vi "State Logic.vi"(0 "TLB' data in":refnum<class "Synchronize AWS S3 Content TLB`.lvclass">, 1 "process state logic enable":bool, 5 "trigger queue in":refnum<queue>, 7 "action queue in":refnum<queue>, 11 "error in":errorcluster) -> (4 "TLB' data out":refnum<class "Synchronize AWS S3 Content TLB`.lvclass">, 15 "error out":errorcluster)   [LabVIEW 2026, in "Synchronize AWS S3 Content.lvlib" / "Synchronize AWS S3 Content TLB`.lvclass"]
doc: "Control process for TLB' template.\n\n<B>Input Parameters</B>\n\n<B>TLB' data in</B> is the templates' private data.\n\n<B>process state logic enable</B> enable state logic change.\n\n<B>trigger queue in</B> is a reference to a queue. Use the Create Trigger Queue function to obtain a queue reference. \n\n<B>action queue in</B> is a reference to a queue. Use the Create Action Queue function to obtain a queue reference. \n\n<B>timeout (ms)</B> queue timeout.\n\n<B>error in</B> describes error conditions that occur before this node runs. This input provides standard error in functionality.\n\n<B>Output Parameters</B>\n\n<B>TLB' data out</B> is the templates' private data.\n\n<B>error out</B> contains error information. This output provides standard error out functionality."
uses:
  Synchronize AWS S3 Content TLB`.lvclass
  Application Components/Trigger API/System Trigger Element.ctl
  Application Components/Trigger API/System Trigger.ctl
  Core Components/Actions/System Action Element.ctl
  Synchronize AWS S3 Content TLB`.lvclass/Synchronize AWS S3 Content TLB`.ctl
  State.ctl
  Core Components/Error Handler/TLB` Error Handler.lvclass/TLB` Error Handler.ctl
  Core Components/Error Handler/accessors/Get Action Causing Error.vi
  Core Components/Error Handler/accessors/Get Originating State.vi
  Core Components/Error Handler/accessors/Get Destination State.vi
  Core Components/Error Handler/accessors/Get Executed System Actions.vi
  Core Components/Error Handler/accessors/Get Remaing System Actions.vi
  Core Components/Error Handler/Core/actions/support/Error FLUSH-LOG-DIALOG.vi
  Core Components/Error Handler/Core/actions/support/Error FLUSH-DIALOG.vi
  Application Components/Trigger API/Synchronize AWS S3 Content Trigger API.lvlib
  Core Components/Error Handler/TLB` Error Handler.lvclass
  Core Components/Actions/Actions.lvlib
  Synchronize AWS S3 Content.lvlib
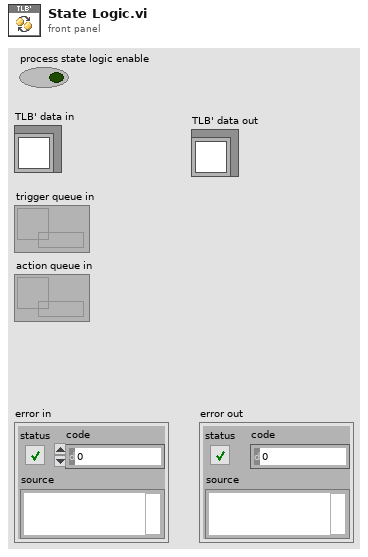
[diagram p1: front panel]
types:
  T1 = typedef "Synchronize AWS S3 Content.lvlib/Synchronize AWS S3 Content TLB`.lvclass/State.ctl" = enum16{"<Startup>", "Idle", "Initiating Configuration", "Validating Commands", "Executing Synchronization", "Validation", "<Shutdown>", "<Error>"}
  T2 = typedef "Synchronize AWS S3 Content.lvlib/Synchronize AWS S3 Content Trigger API.lvlib/System Trigger.ctl" = enum16{"<None>", "<Return to Safe State Actions>", "<Cache User Parameters>", "<Close Application>", "<Error>"}
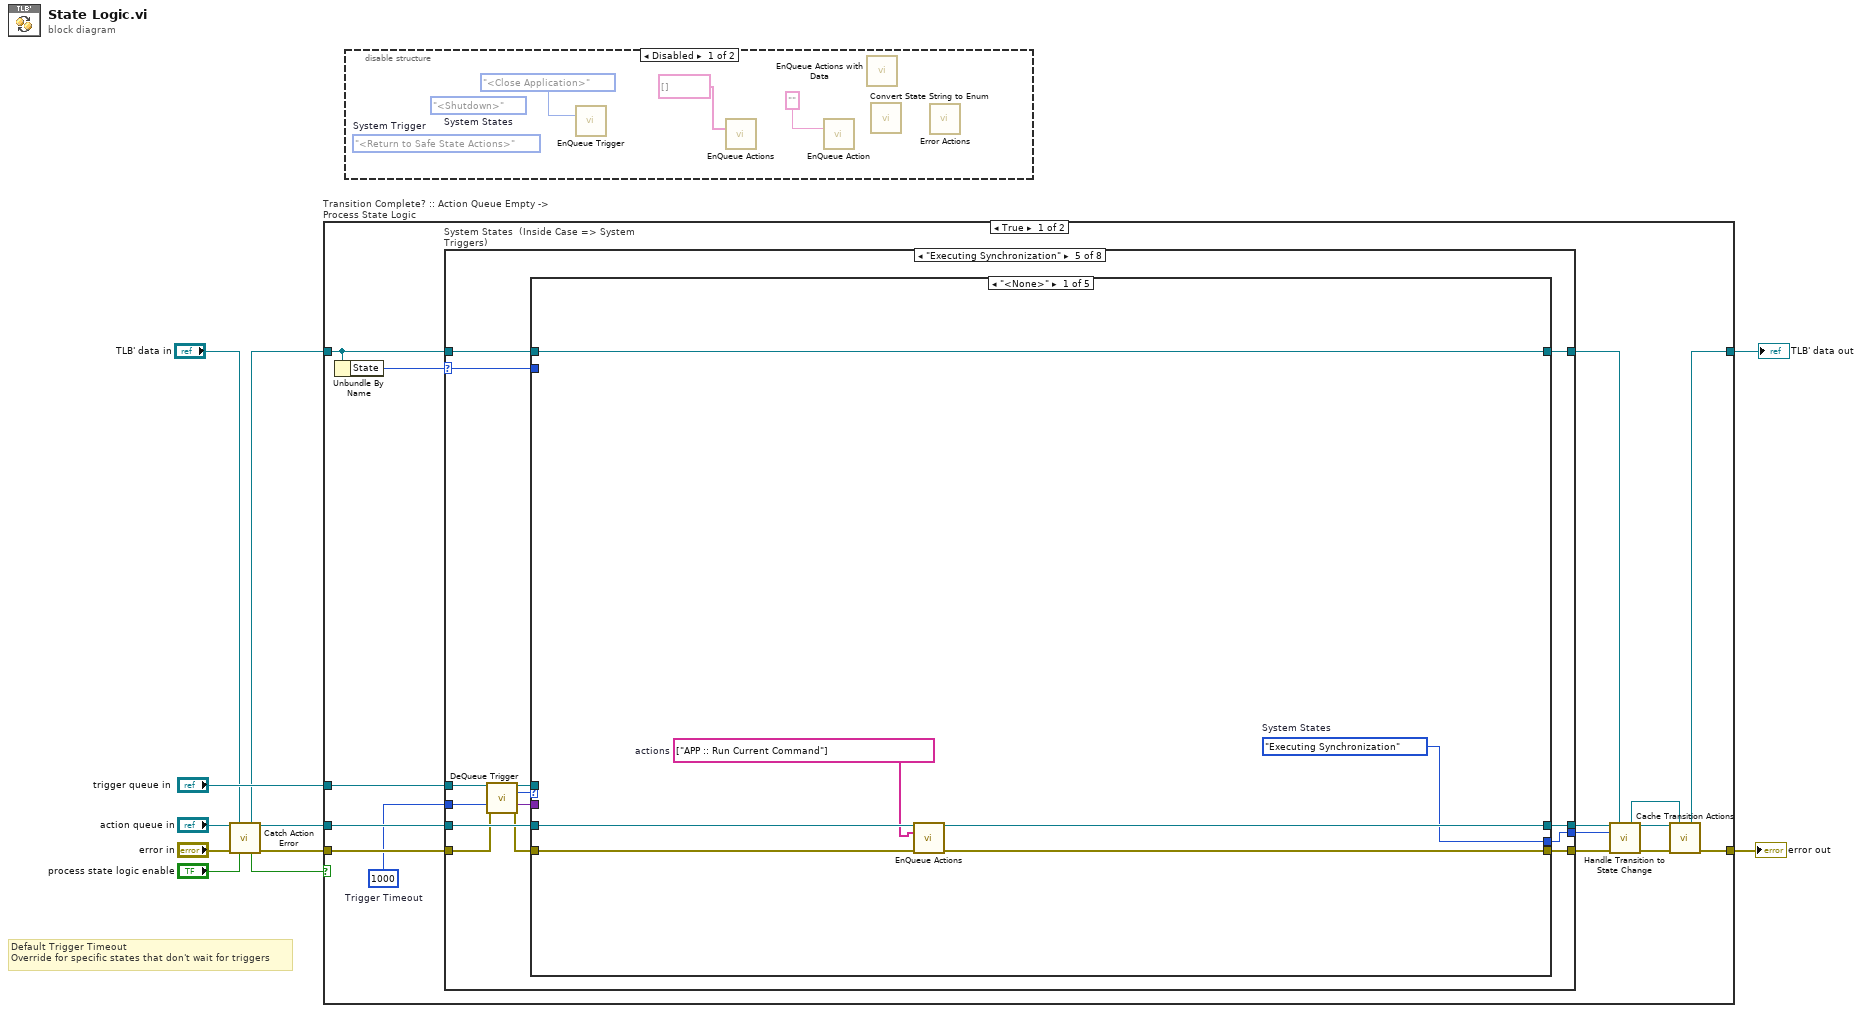
[diagram p0: block diagram]
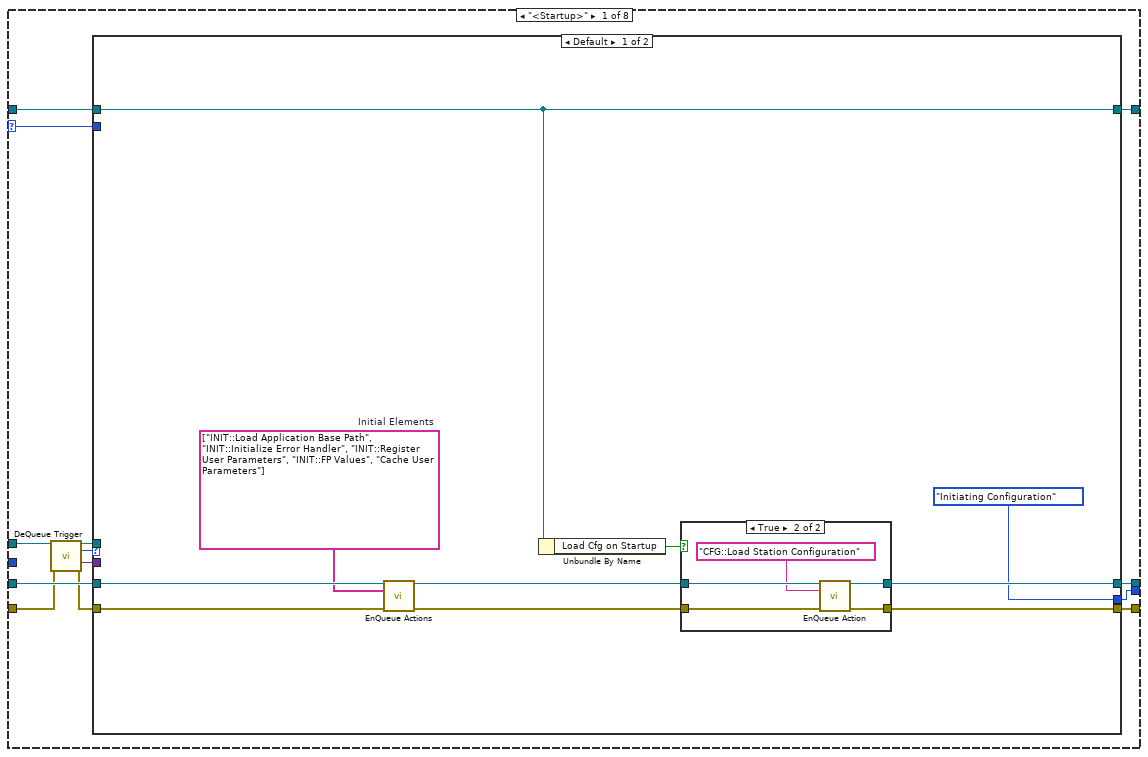
[diagram p3: hidden frame]
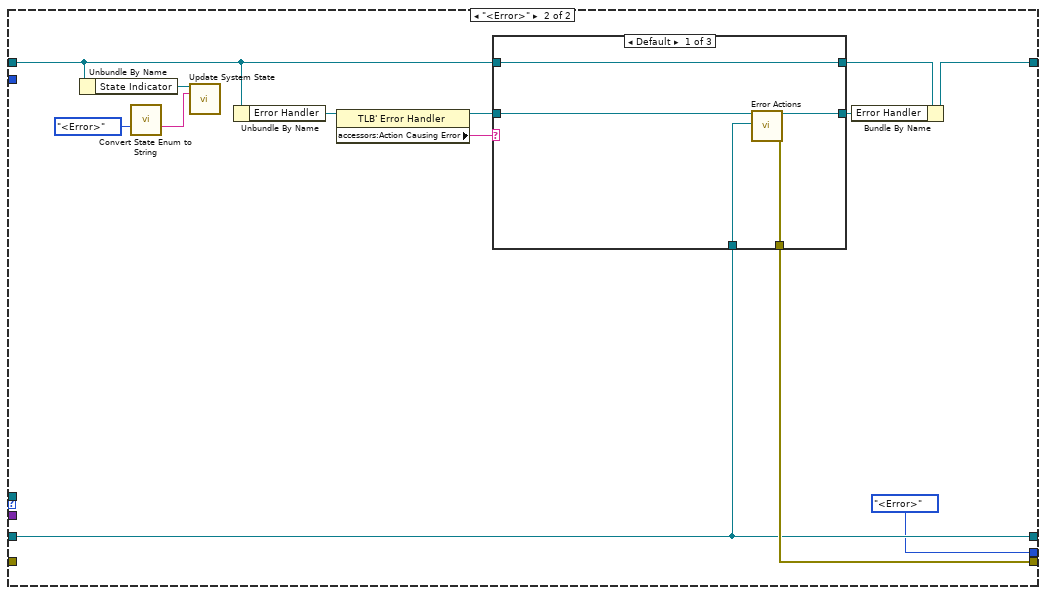
[diagram p5: hidden frame]
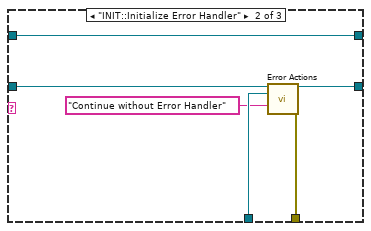
[diagram p6: hidden frame]
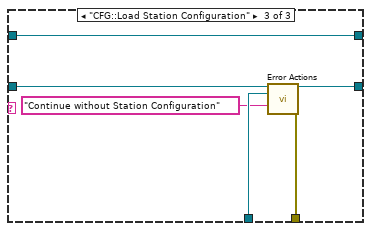
[diagram p7: hidden frame]
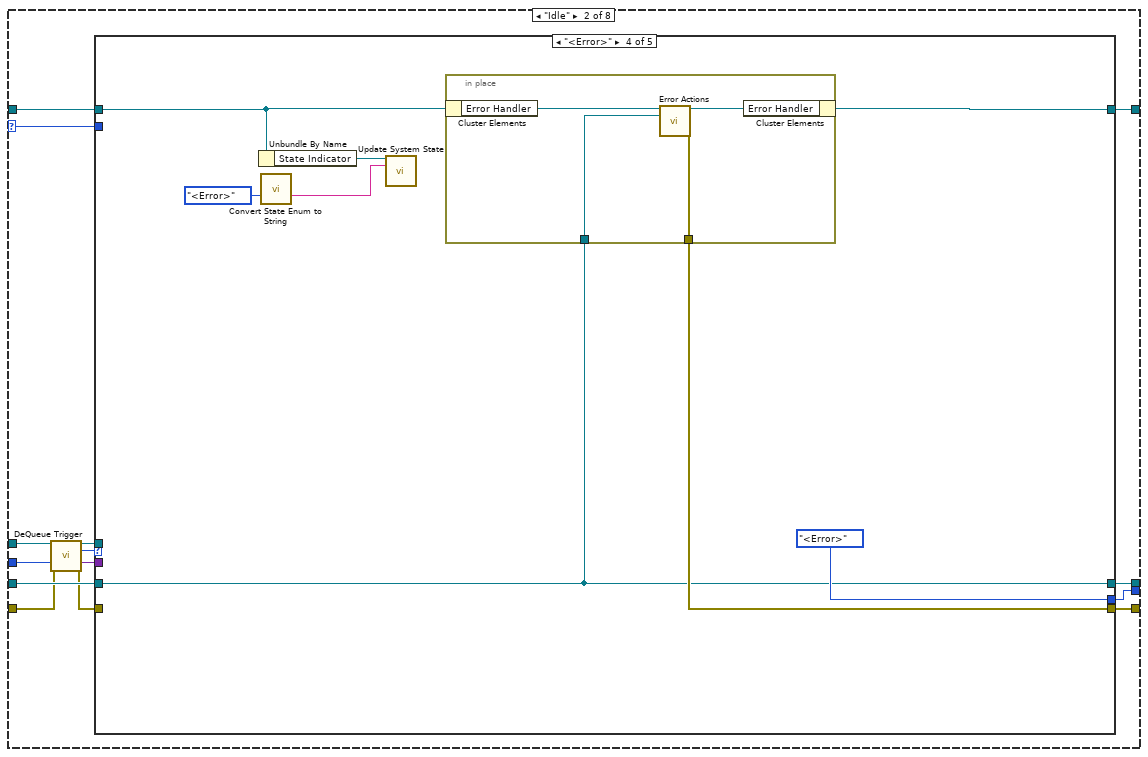
[diagram p8: hidden frame]
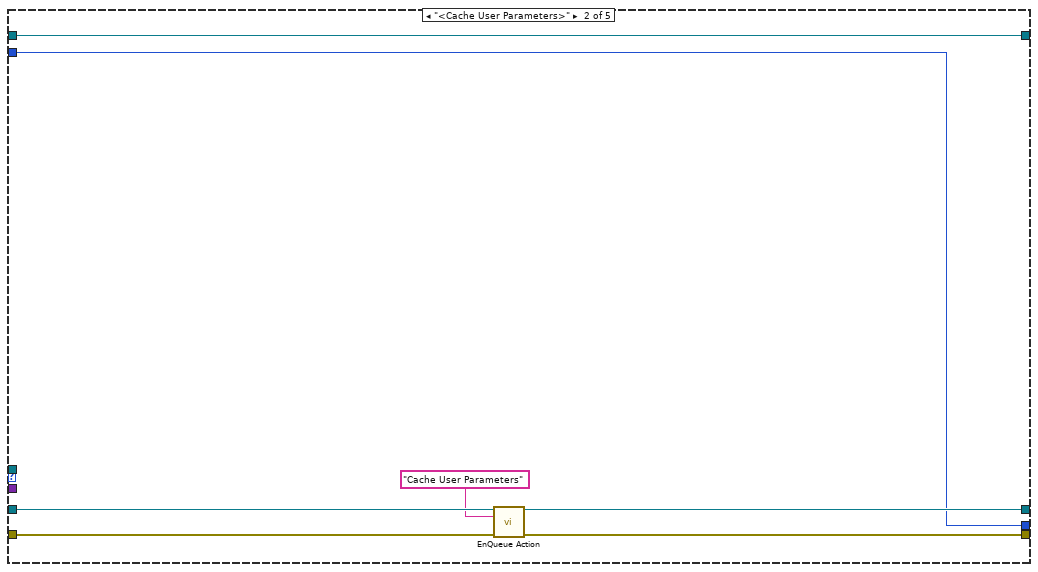
[diagram p10: hidden frame]
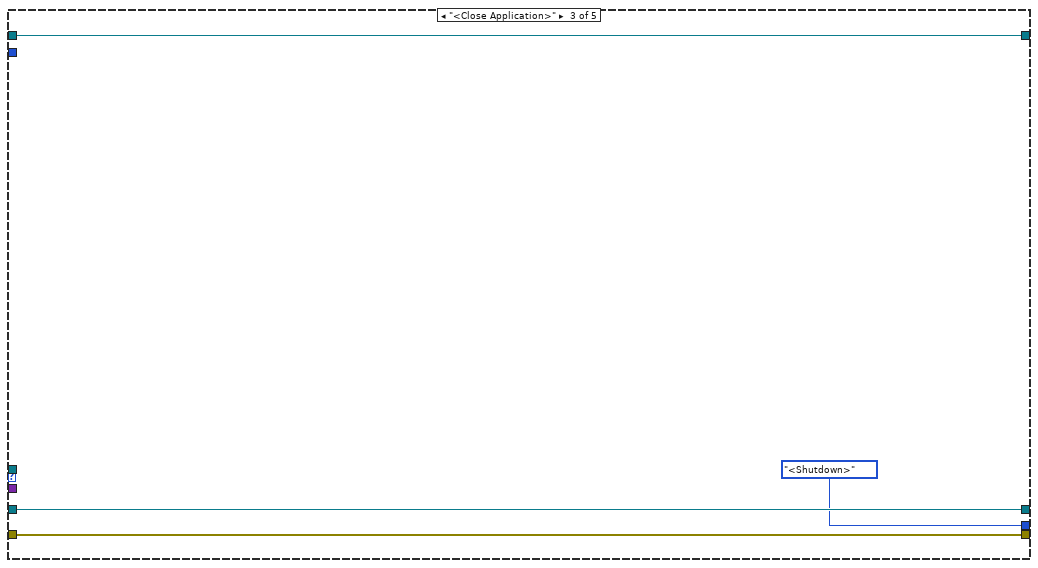
[diagram p11: hidden frame]
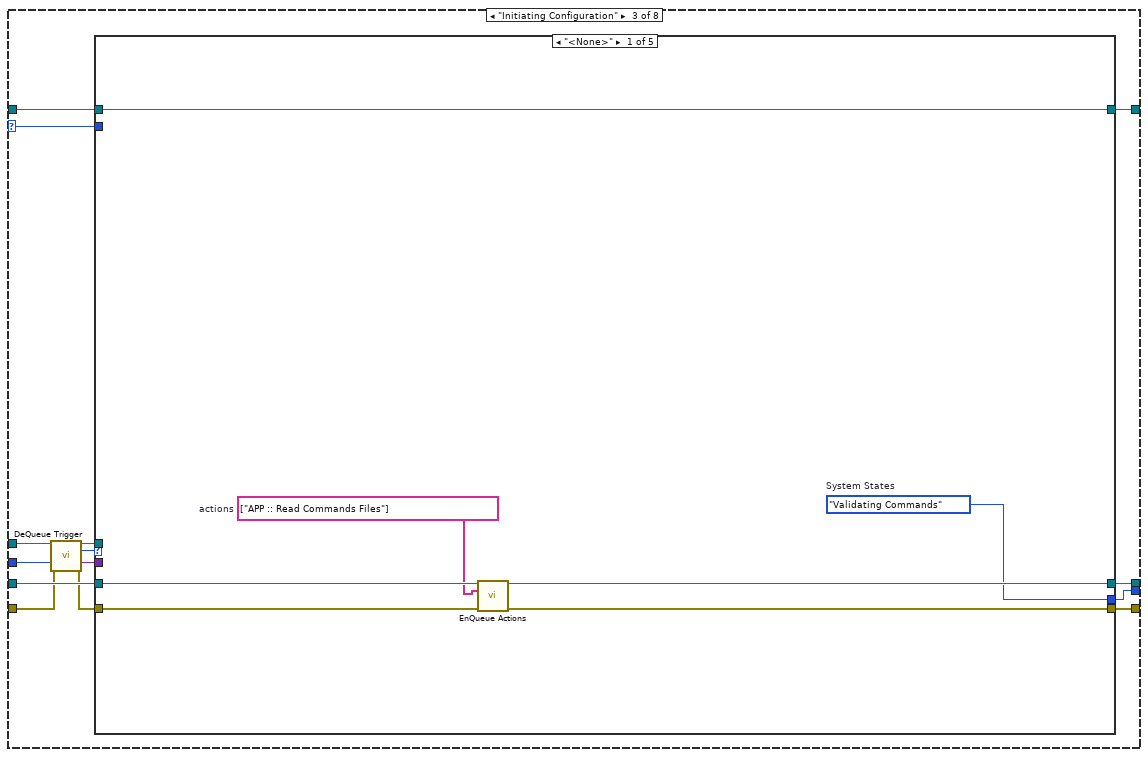
[diagram p13: hidden frame]
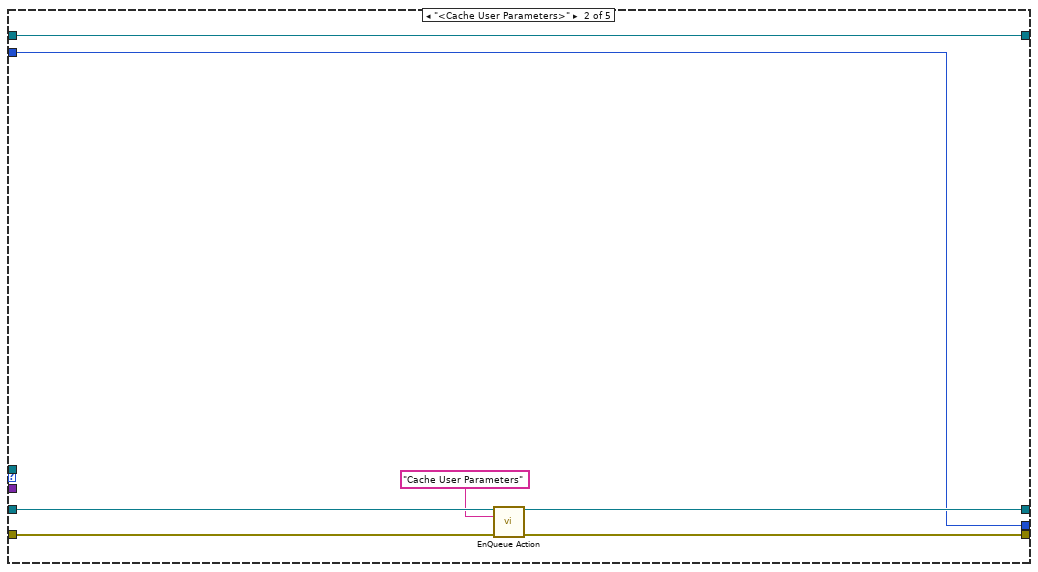
[diagram p14: hidden frame]
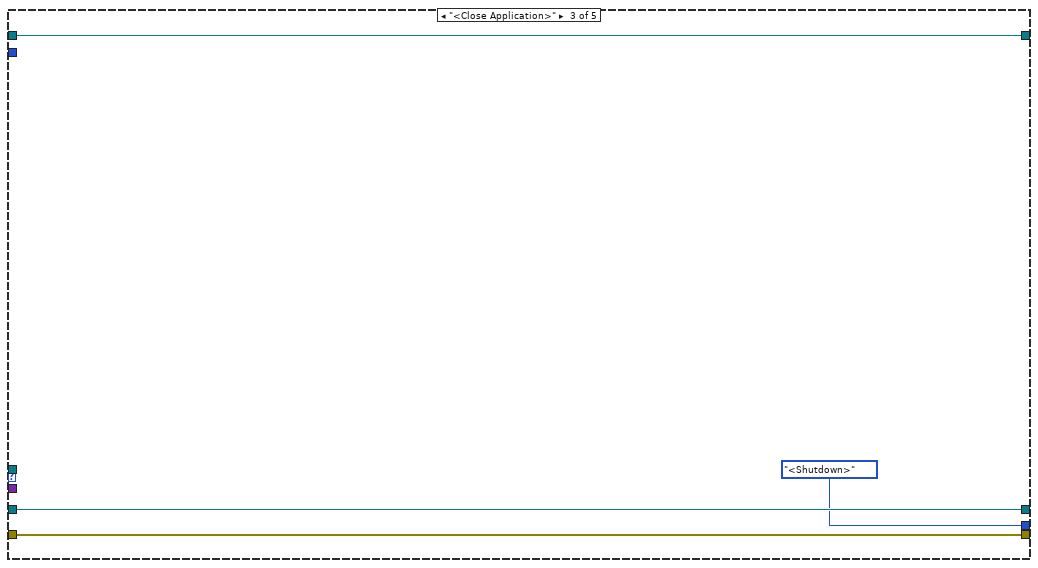
[diagram p15: hidden frame]
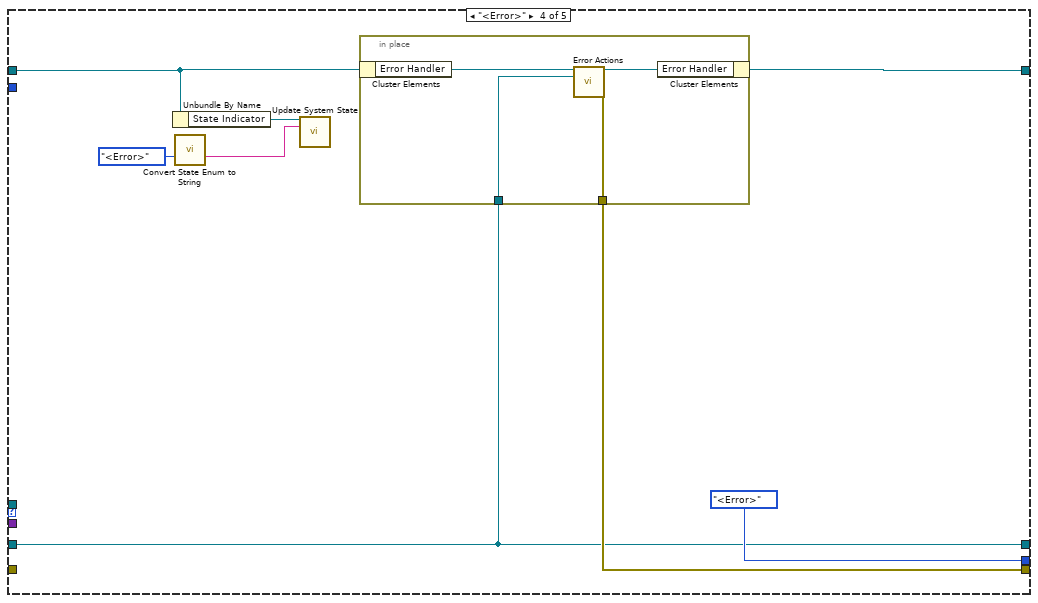
[diagram p16: hidden frame]
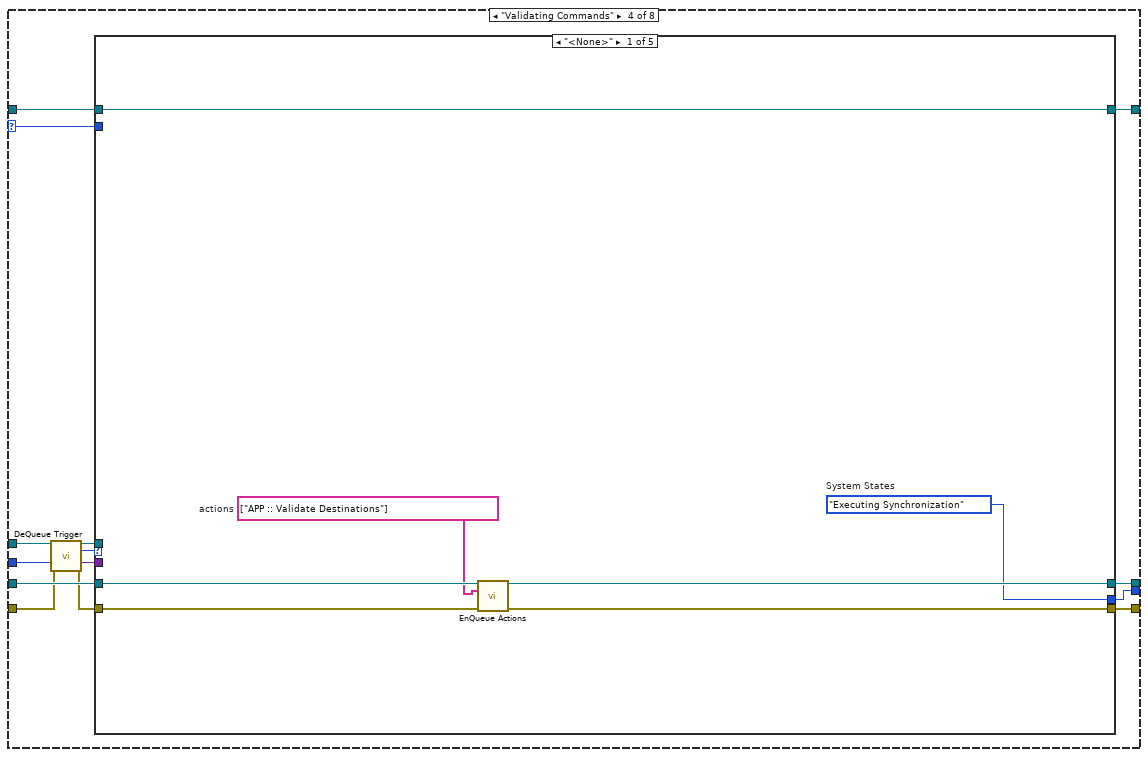
[diagram p18: hidden frame]
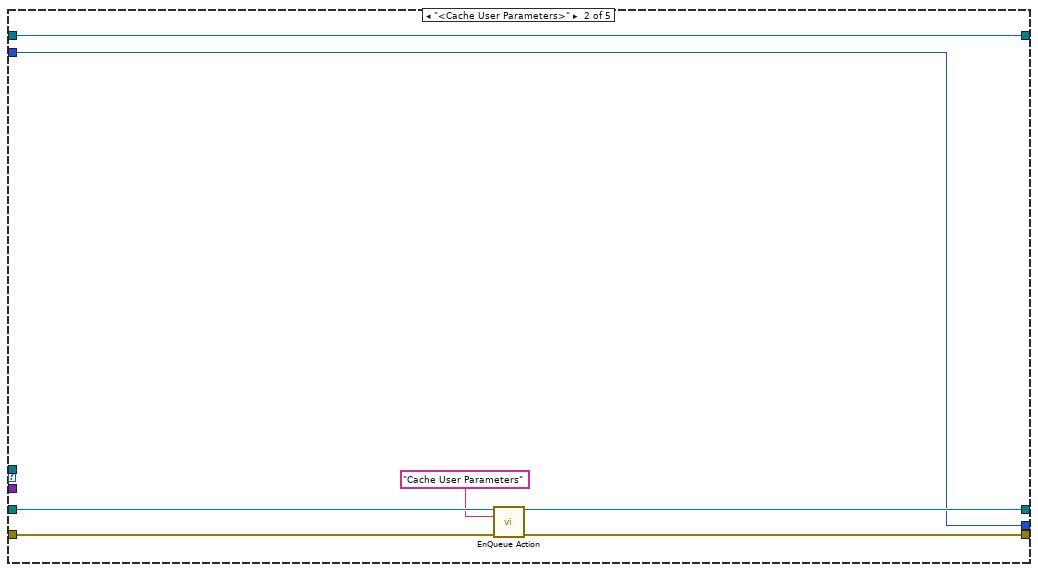
[diagram p19: hidden frame]
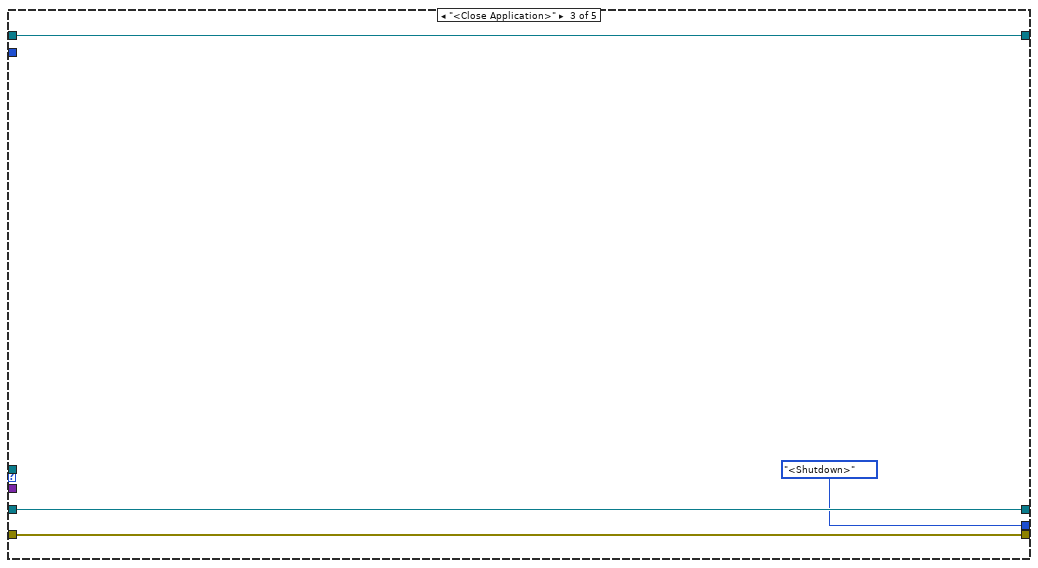
[diagram p20: hidden frame]
diagram:
  # "Default Trigger Timeout\nOverride for specific states that don't wait for triggers"
  n1 = call "Catch Action Error.vi"("action queue in"="action queue in", "TLB' Template in"="TLB' data in", "error in (no error)"="error in", "process state logic enable in"="process state logic enable") -> ("TLB' Template out"=w6:refnum<class "Synchronize AWS S3 Content TLB`.lvclass">, "action queue in"=w2:refnum<queue>, "process state logic enable out"=w4:bool, "error out"=w7:errorcluster)  [unwired: 8 in]
  n2 = case "Transition Complete? :: Action Queue Empty -> Process State Logic" shown="True" w4 {
    tunnel: [w17 w427] -> w10
    tunnel: w6 -> [w22 w427]
    tunnel: w7 -> [w26 w428]
    tunnel: w2 -> [w25 _]
    tunnel: [w20 w428] -> w11
    tunnel: "trigger queue in" -> [w24 _]
    frame True {
      w18 = 1000  # Trigger Timeout
      n3 = Unbundle By Name(w22) -> ("State"=w19:T1)
      n4 = case "System States  (Inside Case => System Triggers)" shown="\"Executing Synchronization\"" w19 {
        selector: w19 -> [w27 w89 w134 w182 w230 w278 w328 _]
        tunnel: [w33 w94 w139 w187 w235 w283 w326 w425] -> w15
        tunnel: w22 -> [w34 w95 w140 w188 w236 w284 w327 w425]
        tunnel: w26 -> [w32 w93 w138 w186 w234 w282 w325 w424]
        tunnel: w25 -> [w38 w99 w144 w192 w240 w288 w329 w423]
        tunnel: [w37 w98 w143 w191 w239 w287 w332 w421] -> w23
        tunnel: w24 -> [w39 w100 w145 w193 w241 w289 w333 _]
        tunnel: [w36 w97 w142 w190 w238 w286 w331 w422] -> w16
        tunnel: [w35 w96 w141 w189 w237 w285 w330 State."<Shutdown>" ("State")] -> w12
        tunnel: w18 -> [_ w88 w133 w181 w229 w277 _ _]
        frame "<Startup>" {
          n5 = call "DeQueue Trigger.vi"("trigger queue in"=w39, "error in"=w32) -> ("trigger queue out"=w28:refnum<queue>, "system trigger"=w30:T2, "trigger data"=w29:variant, "error out"=w31:errorcluster)  [unwired: 10 in]
          n6 = case shown="Default" w30 {
            tunnel: w31 -> [w47 _]
            tunnel: w38 -> [w49 w67]
            tunnel: [w44 w68] -> w37
            tunnel: [w42 w67] -> w36
            tunnel: w29 -> [_ _]
            tunnel: [State."Initiating Configuration" ("State") State."<Error>" ("State")] -> w35
            tunnel: w34 -> [w45 w58]
            tunnel: [w45 w69] -> w33
            tunnel: w28 -> [_ _]
            tunnel: w27 -> [_ _]
            frame Default {
              w48 = string[] ["INIT::Load Application Base Path", "INIT::Initialize Error Handler", "INIT::Register User Parameters", "INIT::FP Values", "Cache User Parameters"]  # Initial Elements
              n7 = call "EnQueue Actions.vi"("action queue in"=w49, "actions"=w48, "error in"=w47) -> ("action queue out"=w43:refnum<queue>, "error out"=w46:errorcluster)  [unwired: 11 in]
              n8 = Unbundle By Name(w45) -> ("Load Cfg on Startup"=w41:bool)
              n9 = case shown="True" w41 {
                tunnel: w46 -> [w50 w56]
                tunnel: [w50 w55] -> w44
                tunnel: w43 -> [w51 w54]
                tunnel: [w51 w53] -> w42
                frame False {
                }
                frame True {
                  n10 = call "EnQueue Action.vi"("action queue in"=w54, "action"="CFG::Load Station Configuration", "error in"=w56) -> ("action queue out"=w53:refnum<queue>, "error out"=w55:errorcluster)  [unwired: 11 in]
                }
              }
            }
            frame "<Error>" {
              n11 = Unbundle By Name(w58) -> ("State Indicator"=w62:refnum<user-event>)
              n12 = call "Convert State Enum to String.vi"("state in"=State."<Error>") -> ("state out"=w61:string)  [unwired: 13 in, 1 out]
              n13 = call "Update System State.vi"("State Indicator"=w62, "system state message"=w61) -> ()  [unwired: 13 in, 1 out]
              n14 = Unbundle By Name(w58) -> ("Error Handler"=w64:refnum<class "TLB` Error Handler.lvclass">)
              n15 = property class="TLB' Error Handler"(reference=w64) -> (reference out=w63:refnum<class "TLB` Error Handler.lvclass">, "accessors:Action Causing Error"=w60:string)  [unwired: 1 in, 1 out]
              n16 = case shown="Default" w60 {
                tunnel: [w72 w80 w86] -> w68
                tunnel: w67 -> [w71 w79 w85]
                tunnel: [w73 w78 w84] -> w65
                tunnel: w63 -> [w74 w77 w83]
                tunnel: w58 -> [w70 w75 w81]
                tunnel: [w70 w75 w81] -> w57
                frame Default {
                  n17 = call-poly "Error Actions.vi"("Error Handler in"=w74, "action queue in"=w71) -> ("Error Handler out"=w73:refnum<class "TLB` Error Handler.lvclass">, "error out"=w72:errorcluster)  [unwired: 12 in]
                }
                frame "INIT::Initialize Error Handler" {
                  n18 = call-poly "Error Actions.vi"("Error Handler in"=w77, "action queue in"=w79, "error button text (Return to Safe State)"="Continue without Error Handler") -> ("Error Handler out"=w78:refnum<class "TLB` Error Handler.lvclass">, "error out"=w80:errorcluster)  [unwired: 11 in]
                }
                frame "CFG::Load Station Configuration" {
                  n19 = call-poly "Error Actions.vi"("Error Handler in"=w83, "action queue in"=w85, "error button text (Return to Safe State)"="Continue without Station Configuration") -> ("Error Handler out"=w84:refnum<class "TLB` Error Handler.lvclass">, "error out"=w86:errorcluster)  [unwired: 11 in]
                }
              }
              n20 = Bundle By Name(cluster=w57, "Error Handler"=w65) -> (w69:refnum<class "Synchronize AWS S3 Content TLB`.lvclass">)
            }
          }
        }
        frame "Idle" {
          n21 = call "DeQueue Trigger.vi"("trigger queue in"=w100, "timeout, ms (0)"=w88, "error in"=w93) -> ("trigger queue out"=w87:refnum<queue>, "system trigger"=w91:T2, "trigger data"=w90:variant, "error out"=w92:errorcluster)  [unwired: 9 in]
          n22 = case shown="\"<Error>\"" w91 {
            tunnel: w92 -> [w103 w111 w114 _ w130]
            tunnel: w99 -> [w104 w108 w115 w119 w131]
            tunnel: [w103 w109 w114 w121 w130] -> w98
            tunnel: [w104 w107 w115 w119 w131] -> w97
            tunnel: w90 -> [_ _ _ _ _]
            tunnel: w95 -> [w102 w110 w113 w118 w129]
            tunnel: [w101 w105 State."<Shutdown>" ("State") State."<Error>" ("State") w128] -> w96
            tunnel: [w102 w110 w113 w120 w129] -> w94
            tunnel: w89 -> [w101 w105 _ _ w128]
            tunnel: w87 -> [_ _ _ _ _]
            frame "<None>" {
            }
            frame "<Cache User Parameters>" {
              n23 = call "EnQueue Action.vi"("action queue in"=w108, "action"="Cache User Parameters", "error in"=w111) -> ("action queue out"=w107:refnum<queue>, "error out"=w109:errorcluster)  [unwired: 11 in]
            }
            frame "<Close Application>" {
            }
            frame "<Error>" {
              n24 = Unbundle By Name(w118) -> ("State Indicator"=w122:refnum<user-event>)
              n25 = call "Convert State Enum to String.vi"("state in"=State."<Error>") -> ("state out"=w116:string)  [unwired: 13 in, 1 out]
              n26 = call "Update System State.vi"("State Indicator"=w122, "system state message"=w116) -> ()  [unwired: 13 in, 1 out]
              n27 = in-place {
                in-place-border: [w125] -> w121
                in-place-border: w119 -> [w124]
                n28 = in-place-cluster #1(w118) -> ("Error Handler"=w127:refnum<class "TLB` Error Handler.lvclass">)
                n29 = call-poly "Error Actions.vi"("Error Handler in"=w127, "action queue in"=w124) -> ("Error Handler out"=w126:refnum<class "TLB` Error Handler.lvclass">, "error out"=w125:errorcluster)  [unwired: 12 in]
                n30 = in-place-cluster #1("Error Handler"=w126) -> (w120:refnum<class "Synchronize AWS S3 Content TLB`.lvclass">)
              }
            }
            frame Default {
            }
          }
        }
        frame "Initiating Configuration" {
          n31 = call "DeQueue Trigger.vi"("trigger queue in"=w145, "timeout, ms (0)"=w133, "error in"=w138) -> ("trigger queue out"=w132:refnum<queue>, "system trigger"=w136:T2, "trigger data"=w135:variant, "error out"=w137:errorcluster)  [unwired: 9 in]
          n32 = case shown="\"<None>\"" w136 {
            tunnel: w137 -> [w152 w159 w162 _ w178]
            tunnel: w144 -> [w149 w156 w163 w167 w179]
            tunnel: [w150 w157 w162 w169 w178] -> w143
            tunnel: [w148 w155 w163 w167 w179] -> w142
            tunnel: w135 -> [_ _ _ _ _]
            tunnel: w140 -> [w151 w158 w161 w166 w177]
            tunnel: [w146 w153 State."<Shutdown>" ("State") State."<Error>" ("State") w176] -> w141
            tunnel: [w151 w158 w161 w168 w177] -> w139
            tunnel: w134 -> [_ w153 _ _ w176]
            tunnel: w132 -> [_ _ _ _ _]
            frame "<None>" {
              w146 = State."Validating Commands"  # System States
              w147 = string[] ["APP :: Read Commands Files"]  # actions
              n33 = call "EnQueue Actions.vi"("action queue in"=w149, "actions"=w147, "error in"=w152) -> ("action queue out"=w148:refnum<queue>, "error out"=w150:errorcluster)  [unwired: 11 in]
            }
            frame "<Cache User Parameters>" {
              n34 = call "EnQueue Action.vi"("action queue in"=w156, "action"="Cache User Parameters", "error in"=w159) -> ("action queue out"=w155:refnum<queue>, "error out"=w157:errorcluster)  [unwired: 11 in]
            }
            frame "<Close Application>" {
            }
            frame "<Error>" {
              n35 = Unbundle By Name(w166) -> ("State Indicator"=w170:refnum<user-event>)
              n36 = call "Convert State Enum to String.vi"("state in"=State."<Error>") -> ("state out"=w164:string)  [unwired: 13 in, 1 out]
              n37 = call "Update System State.vi"("State Indicator"=w170, "system state message"=w164) -> ()  [unwired: 13 in, 1 out]
              n38 = in-place {
                in-place-border: [w173] -> w169
                in-place-border: w167 -> [w172]
                n39 = in-place-cluster #2(w166) -> ("Error Handler"=w175:refnum<class "TLB` Error Handler.lvclass">)
                n40 = call-poly "Error Actions.vi"("Error Handler in"=w175, "action queue in"=w172) -> ("Error Handler out"=w174:refnum<class "TLB` Error Handler.lvclass">, "error out"=w173:errorcluster)  [unwired: 12 in]
                n41 = in-place-cluster #2("Error Handler"=w174) -> (w168:refnum<class "Synchronize AWS S3 Content TLB`.lvclass">)
              }
            }
            frame Default {
            }
          }
        }
        frame "Validating Commands" {
          n42 = call "DeQueue Trigger.vi"("trigger queue in"=w193, "timeout, ms (0)"=w181, "error in"=w186) -> ("trigger queue out"=w180:refnum<queue>, "system trigger"=w184:T2, "trigger data"=w183:variant, "error out"=w185:errorcluster)  [unwired: 9 in]
          n43 = case shown="\"<None>\"" w184 {
            tunnel: w185 -> [w200 w207 w210 _ w226]
            tunnel: w192 -> [w197 w204 w211 w215 w227]
            tunnel: [w198 w205 w210 w217 w226] -> w191
            tunnel: [w196 w203 w211 w215 w227] -> w190
            tunnel: w183 -> [_ _ _ _ _]
            tunnel: w188 -> [w199 w206 w209 w214 w225]
            tunnel: [w194 w201 State."<Shutdown>" ("State") State."<Error>" ("State") w224] -> w189
            tunnel: [w199 w206 w209 w216 w225] -> w187
            tunnel: w182 -> [_ w201 _ _ w224]
            tunnel: w180 -> [_ _ _ _ _]
            frame "<None>" {
              w194 = State."Executing Synchronization"  # System States
              w195 = string[] ["APP :: Validate Destinations"]  # actions
              n44 = call "EnQueue Actions.vi"("action queue in"=w197, "actions"=w195, "error in"=w200) -> ("action queue out"=w196:refnum<queue>, "error out"=w198:errorcluster)  [unwired: 11 in]
            }
            frame "<Cache User Parameters>" {
              n45 = call "EnQueue Action.vi"("action queue in"=w204, "action"="Cache User Parameters", "error in"=w207) -> ("action queue out"=w203:refnum<queue>, "error out"=w205:errorcluster)  [unwired: 11 in]
            }
            frame "<Close Application>" {
            }
            frame "<Error>" {
              n46 = Unbundle By Name(w214) -> ("State Indicator"=w218:refnum<user-event>)
              n47 = call "Convert State Enum to String.vi"("state in"=State."<Error>") -> ("state out"=w212:string)  [unwired: 13 in, 1 out]
              n48 = call "Update System State.vi"("State Indicator"=w218, "system state message"=w212) -> ()  [unwired: 13 in, 1 out]
              n49 = in-place {
                in-place-border: [w221] -> w217
                in-place-border: w215 -> [w220]
                n50 = in-place-cluster #3(w214) -> ("Error Handler"=w223:refnum<class "TLB` Error Handler.lvclass">)
                n51 = call-poly "Error Actions.vi"("Error Handler in"=w223, "action queue in"=w220) -> ("Error Handler out"=w222:refnum<class "TLB` Error Handler.lvclass">, "error out"=w221:errorcluster)  [unwired: 12 in]
                n52 = in-place-cluster #3("Error Handler"=w222) -> (w216:refnum<class "Synchronize AWS S3 Content TLB`.lvclass">)
              }
            }
            frame Default {
            }
          }
        }
        frame "Executing Synchronization" {
          n53 = call "DeQueue Trigger.vi"("trigger queue in"=w241, "timeout, ms (0)"=w229, "error in"=w234) -> ("trigger queue out"=w228:refnum<queue>, "system trigger"=w232:T2, "trigger data"=w231:variant, "error out"=w233:errorcluster)  [unwired: 9 in]
          n54 = case shown="\"<None>\"" w232 {
            tunnel: w233 -> [w248 w255 w258 _ w274]
            tunnel: w240 -> [w245 w252 w259 w263 w275]
            tunnel: [w246 w253 w258 w265 w274] -> w239
            tunnel: [w244 w251 w259 w263 w275] -> w238
            tunnel: w231 -> [_ _ _ _ _]
            tunnel: w236 -> [w247 w254 w257 w262 w273]
            tunnel: [w242 w249 State."<Shutdown>" ("State") State."<Error>" ("State") w272] -> w237
            tunnel: [w247 w254 w257 w264 w273] -> w235
            tunnel: w230 -> [_ w249 _ _ w272]
            tunnel: w228 -> [_ _ _ _ _]
            frame "<None>" {
              w242 = State."Executing Synchronization"  # System States
              w243 = string[] ["APP :: Run Current Command"]  # actions
              n55 = call "EnQueue Actions.vi"("action queue in"=w245, "actions"=w243, "error in"=w248) -> ("action queue out"=w244:refnum<queue>, "error out"=w246:errorcluster)  [unwired: 11 in]
            }
            frame "<Cache User Parameters>" {
              n56 = call "EnQueue Action.vi"("action queue in"=w252, "action"="Cache User Parameters", "error in"=w255) -> ("action queue out"=w251:refnum<queue>, "error out"=w253:errorcluster)  [unwired: 11 in]
            }
            frame "<Close Application>" {
            }
            frame "<Error>" {
              n57 = Unbundle By Name(w262) -> ("State Indicator"=w266:refnum<user-event>)
              n58 = call "Convert State Enum to String.vi"("state in"=State."<Error>") -> ("state out"=w260:string)  [unwired: 13 in, 1 out]
              n59 = call "Update System State.vi"("State Indicator"=w266, "system state message"=w260) -> ()  [unwired: 13 in, 1 out]
              n60 = in-place {
                in-place-border: [w269] -> w265
                in-place-border: w263 -> [w268]
                n61 = in-place-cluster #4(w262) -> ("Error Handler"=w271:refnum<class "TLB` Error Handler.lvclass">)
                n62 = call-poly "Error Actions.vi"("Error Handler in"=w271, "action queue in"=w268) -> ("Error Handler out"=w270:refnum<class "TLB` Error Handler.lvclass">, "error out"=w269:errorcluster)  [unwired: 12 in]
                n63 = in-place-cluster #4("Error Handler"=w270) -> (w264:refnum<class "Synchronize AWS S3 Content TLB`.lvclass">)
              }
            }
            frame Default {
            }
          }
        }
        frame "Validation" {
          n64 = call "DeQueue Trigger.vi"("trigger queue in"=w289, "timeout, ms (0)"=w277, "error in"=w282) -> ("trigger queue out"=w276:refnum<queue>, "system trigger"=w280:T2, "trigger data"=w279:variant, "error out"=w281:errorcluster)  [unwired: 9 in]
          n65 = case shown="\"<None>\"" w280 {
            tunnel: w281 -> [w292 w300 w303 _ w319]
            tunnel: w288 -> [w293 w297 w304 w308 w320]
            tunnel: [w292 w298 w303 w310 w319] -> w287
            tunnel: [w293 w296 w304 w308 w320] -> w286
            tunnel: w279 -> [_ _ _ _ _]
            tunnel: w284 -> [w291 w299 w302 w307 w318]
            tunnel: [w290 w294 State."<Shutdown>" ("State") State."<Error>" ("State") w317] -> w285
            tunnel: [w291 w299 w302 w309 w318] -> w283
            tunnel: w278 -> [w290 w294 _ _ w317]
            tunnel: w276 -> [_ _ _ _ _]
            frame "<None>" {
            }
            frame "<Cache User Parameters>" {
              n66 = call "EnQueue Action.vi"("action queue in"=w297, "action"="Cache User Parameters", "error in"=w300) -> ("action queue out"=w296:refnum<queue>, "error out"=w298:errorcluster)  [unwired: 11 in]
            }
            frame "<Close Application>" {
            }
            frame "<Error>" {
              n67 = Unbundle By Name(w307) -> ("State Indicator"=w311:refnum<user-event>)
              n68 = call "Convert State Enum to String.vi"("state in"=State."<Error>") -> ("state out"=w305:string)  [unwired: 13 in, 1 out]
              n69 = call "Update System State.vi"("State Indicator"=w311, "system state message"=w305) -> ()  [unwired: 13 in, 1 out]
              n70 = in-place {
                in-place-border: [w314] -> w310
                in-place-border: w308 -> [w313]
                n71 = in-place-cluster #5(w307) -> ("Error Handler"=w316:refnum<class "TLB` Error Handler.lvclass">)
                n72 = call-poly "Error Actions.vi"("Error Handler in"=w316, "action queue in"=w313) -> ("Error Handler out"=w315:refnum<class "TLB` Error Handler.lvclass">, "error out"=w314:errorcluster)  [unwired: 12 in]
                n73 = in-place-cluster #5("Error Handler"=w315) -> (w309:refnum<class "Synchronize AWS S3 Content TLB`.lvclass">)
              }
            }
            frame Default {
            }
          }
        }
        frame "<Error>" {
          n74 = call "DeQueue Trigger.vi"("trigger queue in"=w333, "error in"=w325) -> ("trigger queue out"=w324:refnum<queue>, "system trigger"=w323:T2, "trigger data"=w321:variant, "error out"=w322:errorcluster)  [unwired: 10 in]
          n75 = case shown="\"<Close Application>\"" w323 {
            tunnel: w327 -> [w335 w338 w401 w417]
            tunnel: [w336 w348 w410 w416] -> w332
            tunnel: w322 -> [w336 w350 w411 w416]
            tunnel: w329 -> [w337 w351 w412 w419]
            tunnel: [w337 w349 w407 w419] -> w331
            tunnel: [w334 w347 w409 State."<Shutdown>" ("State")] -> w330
            tunnel: w324 -> [_ _ _ _]
            tunnel: w328 -> [w334 _ _ _]
            tunnel: w321 -> [_ _ _ _]
            tunnel: [w335 w346 w401 w417] -> w326
            frame Default {
            }
            frame "<Return to Safe State Actions>" {
              n76 = Unbundle By Name(w338) -> ("Error Handler"=w345:refnum<class "TLB` Error Handler.lvclass">)
              n77 = property class="TLB' Error Handler"(reference=w345) -> ("accessors:Originating State"=w340:string, "accessors:Action Causing Error"=w344:string, "accessors:Destination State"=w343:string, "accessors:Executed System Actions"=w342:string[], "accessors:Remaing System Actions"=w339:string[])  [unwired: 1 in, 2 out]
              n78 = call "Convert State String to Enum.vi"("state in"=w340) -> ("state out"=w341:T1)  [unwired: 13 in, 1 out]
              n79 = case shown="\"<Startup>\"" w341 {
                selector: w341 -> [w352 w359 _]
                tunnel: w351 -> [w355 w365 w398]
                tunnel: w350 -> [w353 w366 w397]
                tunnel: [w353 w364 w397] -> w348
                tunnel: [w355 w363 w398] -> w349
                tunnel: [w352 w362 State."<Shutdown>" ("State")] -> w347
                tunnel: w338 -> [w354 w356 w400]
                tunnel: [w354 w357 w400] -> w346
                tunnel: w344 -> [_ w361 _]
                tunnel: w343 -> [_ w358 _]
                tunnel: w342 -> [_ _ _]
                tunnel: w339 -> [_ w360 _]
                frame Default {
                }
                frame "<Startup>" {
                  n80 = case shown="\"INIT::Initialize Error Handler\"" w361 {
                    tunnel: w366 -> [w369 w382 w395]
                    tunnel: w365 -> [w370 w383 w396]
                    tunnel: [w369 w381 w394] -> w364
                    tunnel: [w370 w380 w393] -> w363
                    tunnel: [State."<Shutdown>" ("State") State."Idle" ("state out") State."Idle" ("state out")] -> w362
                    tunnel: w360 -> [_ w379 w392]
                    tunnel: w359 -> [_ w371 w385]
                    tunnel: w358 -> [_ _ _]
                    tunnel: w356 -> [w367 w373 w386]
                    tunnel: [w367 w372 w384] -> w357
                    frame Default {
                    }
                    frame "INIT::Initialize Error Handler" {
                      n81 = Search 1D Array(1D array=w379, element="Change State") -> (index of element=w377:i32)  [unwired: 1 in]
                      n82 = Delete From Array(array=w379, length=1, index=w377) -> (array with subset deleted=w378:string[])  [unwired: 1 out]
                      n83 = call "EnQueue Actions.vi"("action queue in"=w383, "actions"=w378, "error in"=w382) -> ("action queue out"=w380:refnum<queue>, "error out"=w381:errorcluster)  [unwired: 11 in]
                      n84 = Bundle By Name(cluster=w373, "State"=w371) -> (w372:refnum<class "Synchronize AWS S3 Content TLB`.lvclass">)
                    }
                    frame "CFG::Load Station Configuration" {
                      n85 = Search 1D Array(1D array=w392, element="Change State") -> (index of element=w390:i32)  [unwired: 1 in]
                      n86 = Delete From Array(array=w392, length=1, index=w390) -> (array with subset deleted=w391:string[])  [unwired: 1 out]
                      n87 = call "EnQueue Actions.vi"("action queue in"=w396, "actions"=w391, "error in"=w395) -> ("action queue out"=w393:refnum<queue>, "error out"=w394:errorcluster)  [unwired: 11 in]
                      n88 = Bundle By Name(cluster=w386, "State"=w385) -> (w384:refnum<class "Synchronize AWS S3 Content TLB`.lvclass">)
                    }
                  }
                }
                frame "<Shutdown>" {
                }
              }
            }
            frame "<Close Application>" {
              n89 = Unbundle By Name(w401) -> ("Error Handler"=w408:refnum<class "TLB` Error Handler.lvclass">)
              n90 = property class="TLB' Error Handler"(reference=w408) -> ("accessors:Originating State"=w406:string, "accessors:Action Causing Error"=w402:string, "accessors:Destination State"=w403:string, "accessors:Executed System Actions"=w404:string[])  [unwired: 1 in, 2 out]
              n91 = call "Convert State String to Enum.vi"("state in"=w406) -> ("state out"=w405:T1)  [unwired: 13 in, 1 out]
              n92 = case shown="Default" w405 {
                tunnel: w412 -> [w414]
                tunnel: w411 -> [w413]
                tunnel: [w413] -> w410
                tunnel: [w414] -> w407
                tunnel: [State."<Shutdown>" ("State")] -> w409
                tunnel: w402 -> [_]
                tunnel: w403 -> [_]
                tunnel: w404 -> [_]
                frame Default {
                }
              }
            }
            frame "<Error>" {
              # "If error errors' that is probably really bad and we should end the program"
            }
          }
        }
        frame "<Shutdown>" {
          n93 = call "EnQueue Actions.vi"("action queue in"=w423, "actions"=string[] ["Exit"], "error in"=w424) -> ("action queue out"=w422:refnum<queue>, "error out"=w421:errorcluster)  [unwired: 11 in]
        }
      }
      n94 = call "Handle Transition to State Change.vi"("action queue in"=w16, "TLB' Template in"=w15, "Destination State"=w12, "error in (no error)"=w23) -> ("TLB' Template out"=w14:refnum<class "Synchronize AWS S3 Content TLB`.lvclass">, "action queue in"=w13:refnum<queue>, "error out"=w21:errorcluster)  [unwired: 9 in]
      n95 = call "Cache Transition Actions.vi"("action queue in"=w13, "TLB' Template in"=w14, "error in (no error)"=w21) -> ("TLB' Template out"=w17:refnum<class "Synchronize AWS S3 Content TLB`.lvclass">, "error out"=w20:errorcluster)  [unwired: 11 in]
    }
    frame False {
    }
  }
  "error out" <- w11
  "TLB' data out" <- w10
  n96 = disable-structure shown="Disabled" {
    frame Disabled {
      (unwired) System_Trigger."<Return to Safe State Actions>"  # System Trigger
      (unwired) State."<Shutdown>"  # System States
      n97 = call "EnQueue Trigger.vi"("system trigger"=System_Trigger."<Close Application>" ("System Trigger")) -> ()  [unwired: 13 in, 2 out]
      n98 = call "EnQueue Actions.vi"("actions"=string[] [] ("message names")) -> ()  [unwired: 13 in, 2 out]
      n99 = call "EnQueue Action.vi"("action"="" ("Message Name")) -> ()  [unwired: 13 in, 2 out]
      n100 = call "EnQueue Actions with Data.vi"() -> ()  [unwired: 14 in, 2 out]
      n101 = call "Convert State String to Enum.vi"() -> ()  [unwired: 14 in, 2 out]
      n102 = call-poly "Error Actions.vi"() -> ()  [unwired: 14 in, 2 out]
    }
    frame Enabled {
    }
  }
